vi "configuration UI.vi"() -> ()   [LabVIEW 2013]
uses:
  fixed channel editor.lvclass
  <vilib>/NI/Tag Bus Module Framework/channel/TBM channel.lvclass
  <vilib>/NI/Module Execution Interface/Engine Configuration/engine configuration.lvclass
  <vilib>/NI/Tag Bus/tag/tag descriptor.lvclass
  <vilib>/NI/Configuration Framework/Controls/EventCluster.ctl
  <vilib>/NI/Configuration Framework/NISE_CEF_TreeControl.lvlib
  <vilib>/NI/Tag Bus Data Framework/Configuration Editor/Classes/Engine Parent/Engine Parent Editor Node.lvclass
  <vilib>/NI/Tag Bus Module Framework/module configuration/TBM module configuration.lvclass
  <vilib>/NI/Tag Bus Data Framework/Configuration Editor/Classes/Module editor node/module editor node.lvclass
  module/configuration/fixed channel configuration.lvclass
  <vilib>/NI/Tag Bus Module Framework/channel/channel classification.ctl
  <vilib>/NI/Tools/Keyed Array/KeyedArray.ctl
  <vilib>/NI/Tools/Keyed Array/Tools_KeyedArray.lvlib
  <vilib>/NI/AMC/Message.ctl
  <vilib>/NI/AMC/AMC.lvlib
  <vilib>/NI/AMC/Message Queue.ctl
  <vilib>/NI/Configuration Framework/Node/NISE_CEF_Node.lvclass
  <vilib>/NI/Configuration Framework/Node/NodeRef.ctl
  <vilib>/NI/Configuration Framework/Node/UserEventRef.ctl
panel:
  in  "Tab Control":enum32{"Channels", "Parameters"}(tab)
  in  "mapwriters":bool
  out "Channel List":string[][](table)
  in  "mapall":bool
  in  "kvp":i32(listbox)
  in  "user event":T1
  in  "main queue":T2
  in  "node ref":T3
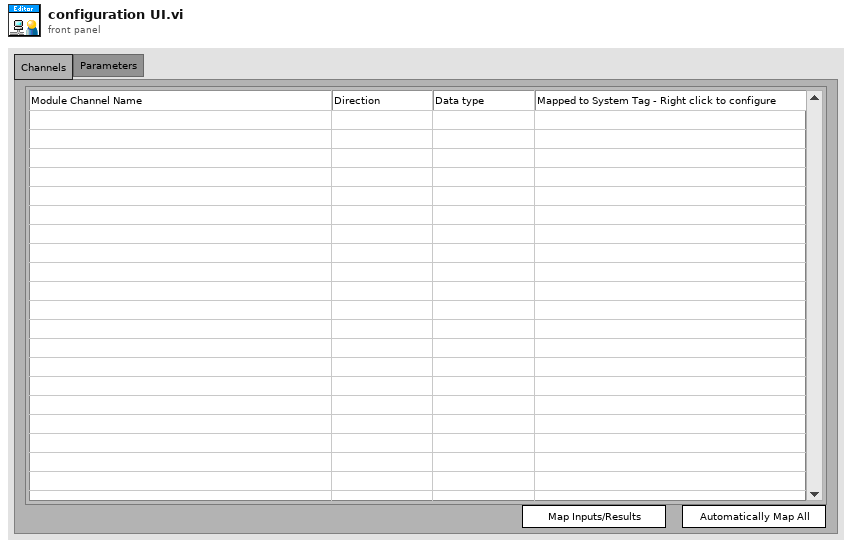
[diagram p1: front panel]
types:
  T1 = typedef "NISE_CEF_Node.lvclass/UserEventRef.ctl" = refnum<user-event>
  T2 = typedef "AMC.lvlib/Message Queue.ctl" = refnum<queue>
  T3 = typedef "NISE_CEF_Node.lvclass/NodeRef.ctl" = refnum<data-value>
  T4 = typedef "NISE_CEF_TreeControl.lvlib/EventCluster.ctl" = cluster{"command":string, "data":string}
  T5 = typedef "LVPoint32TypeDef.ctl" = cluster{"Horizontal":i32, "Vertical":i32}
  T6 = typedef "LVRowAndColumnTypeDef.ctl" = cluster{"Row":i32, "Column":i32}
  T7 = typedef "TBM channel.lvclass/channel classification.ctl" = enum16{"input data", "output data", "processing parameter", "processing result"}
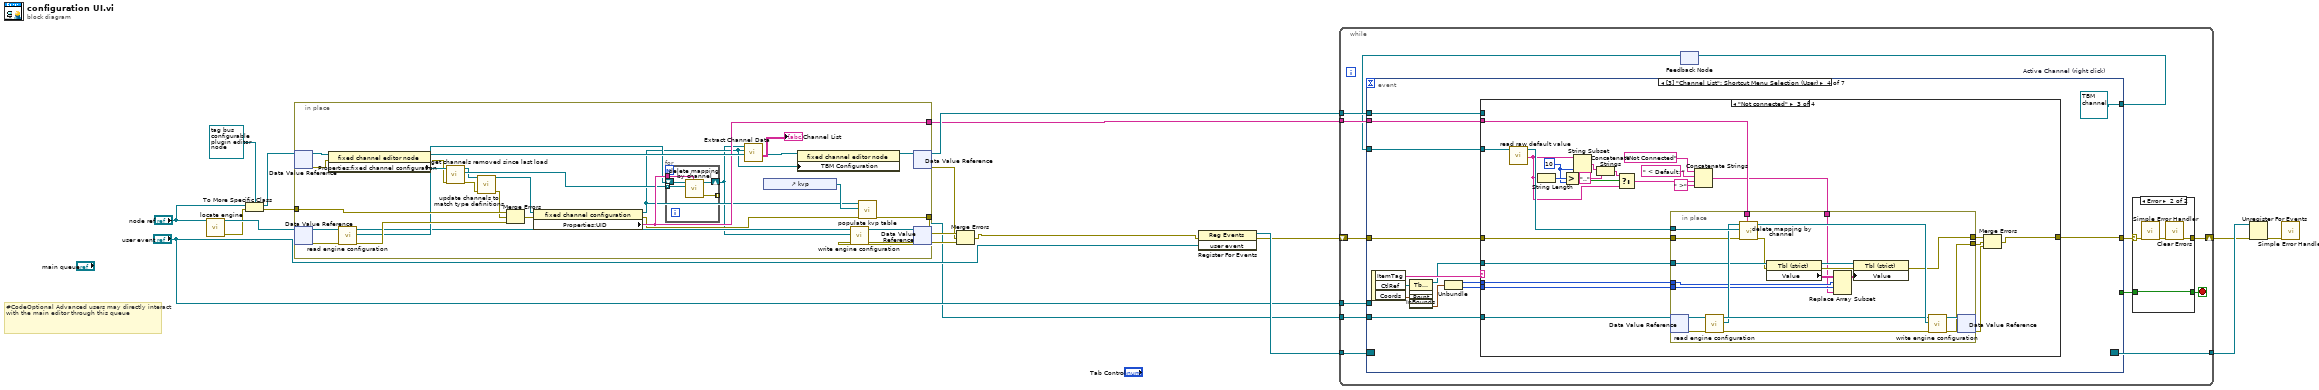
[diagram p0: block diagram]
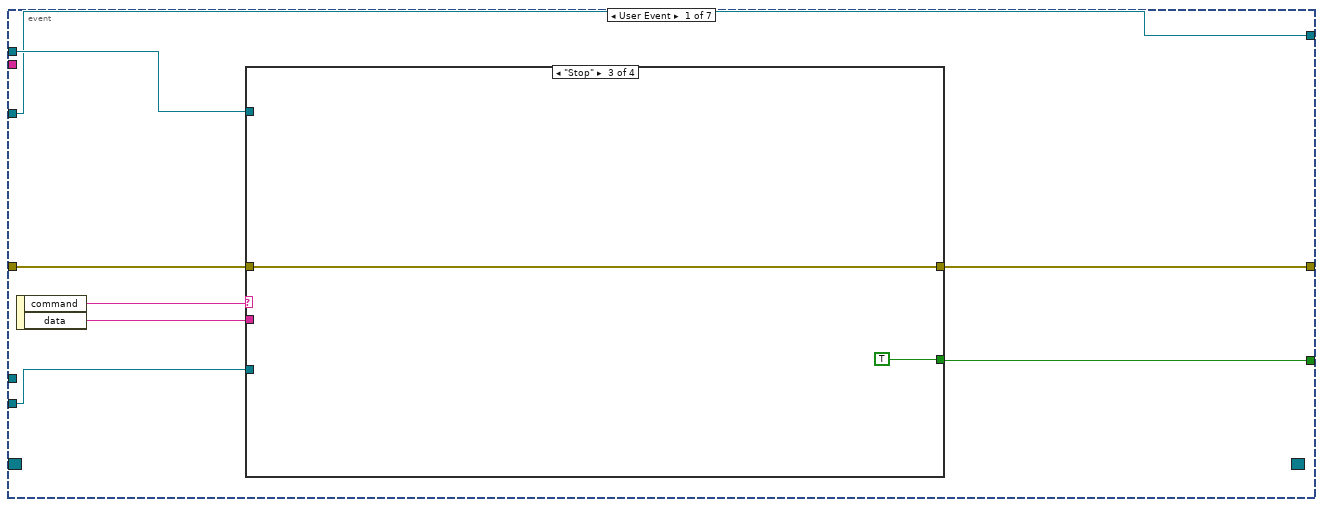
[diagram p3: hidden frame]
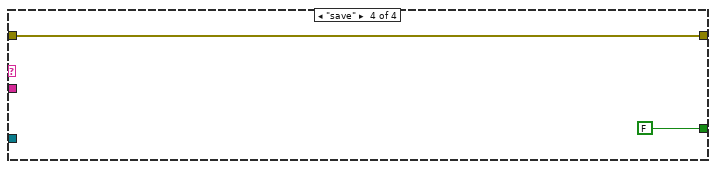
[diagram p6: hidden frame]
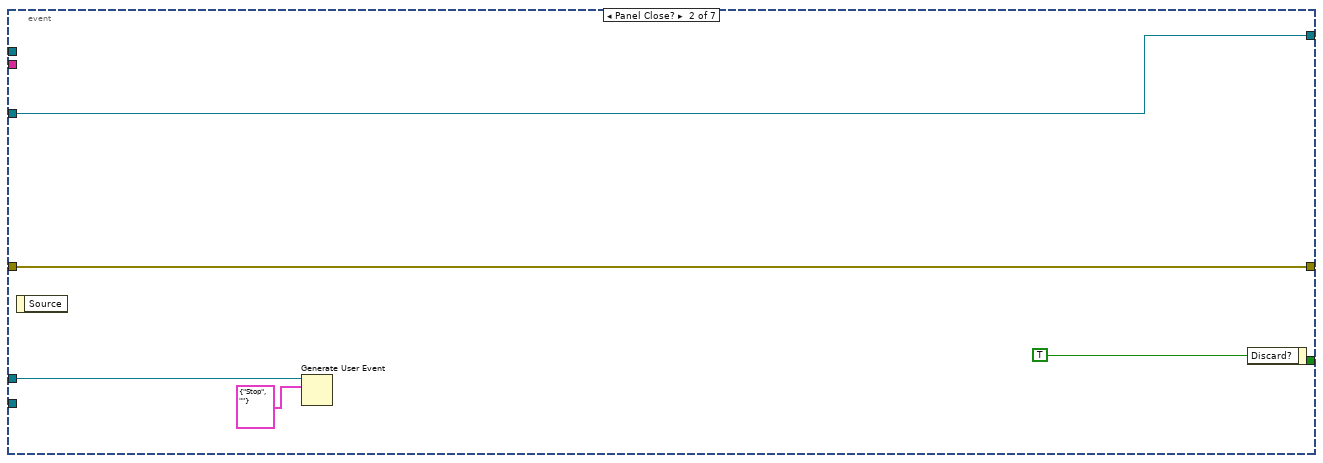
[diagram p7: hidden frame]
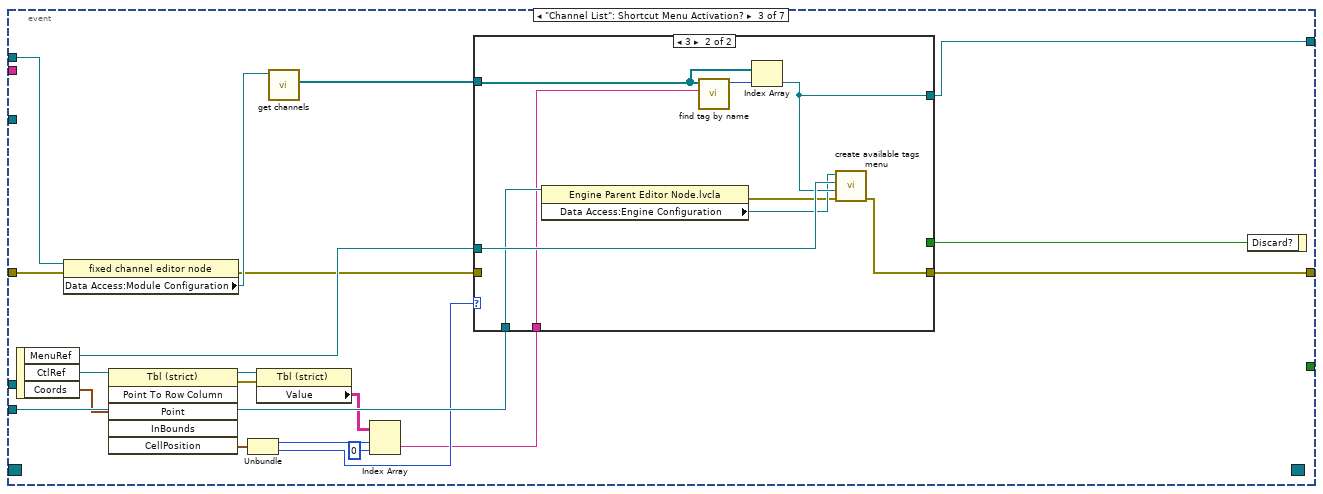
[diagram p8: hidden frame]
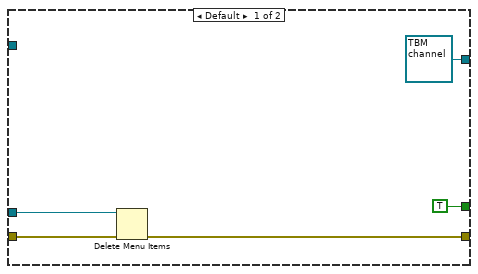
[diagram p9: hidden frame]
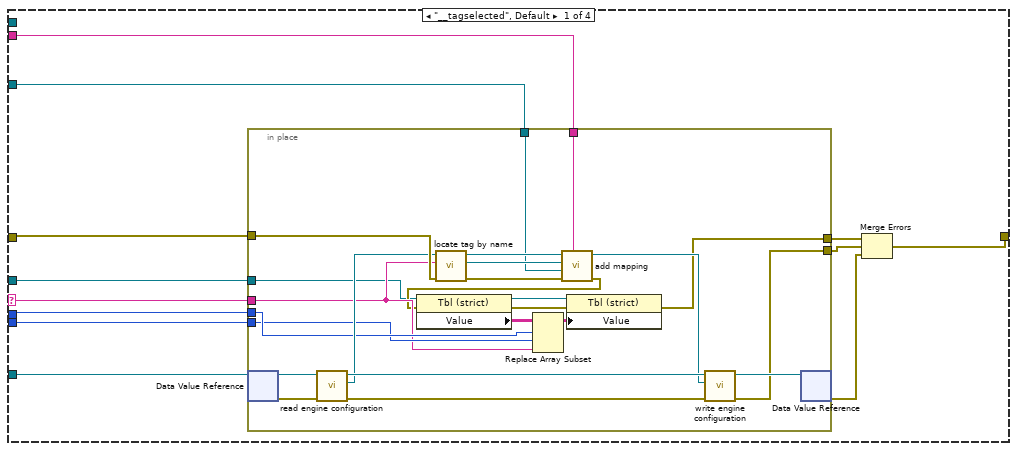
[diagram p10: hidden frame]
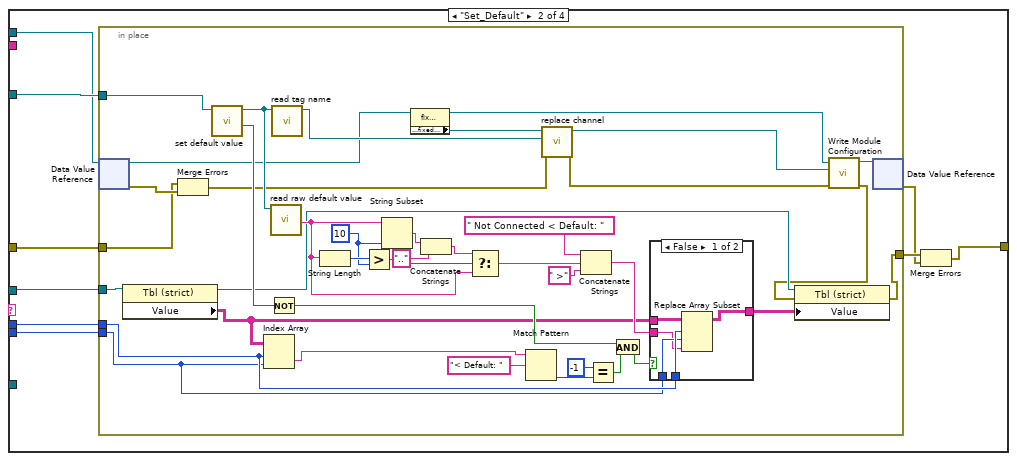
[diagram p11: hidden frame]
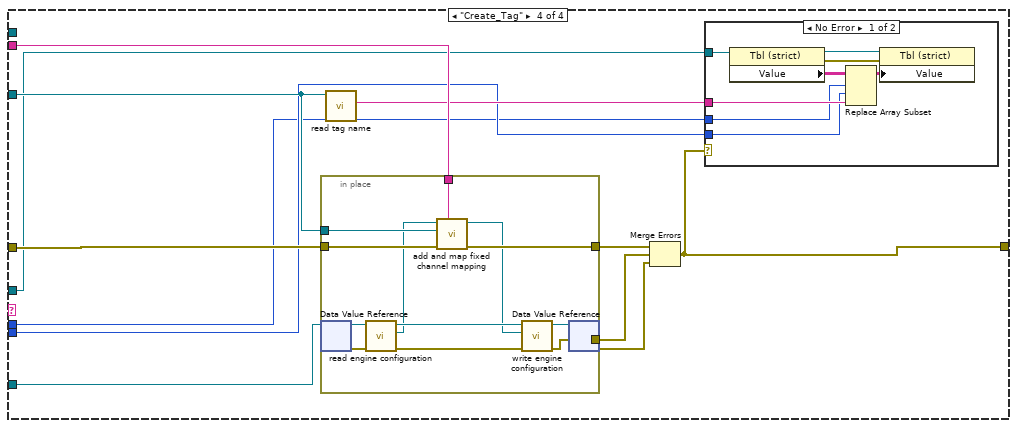
[diagram p13: hidden frame]
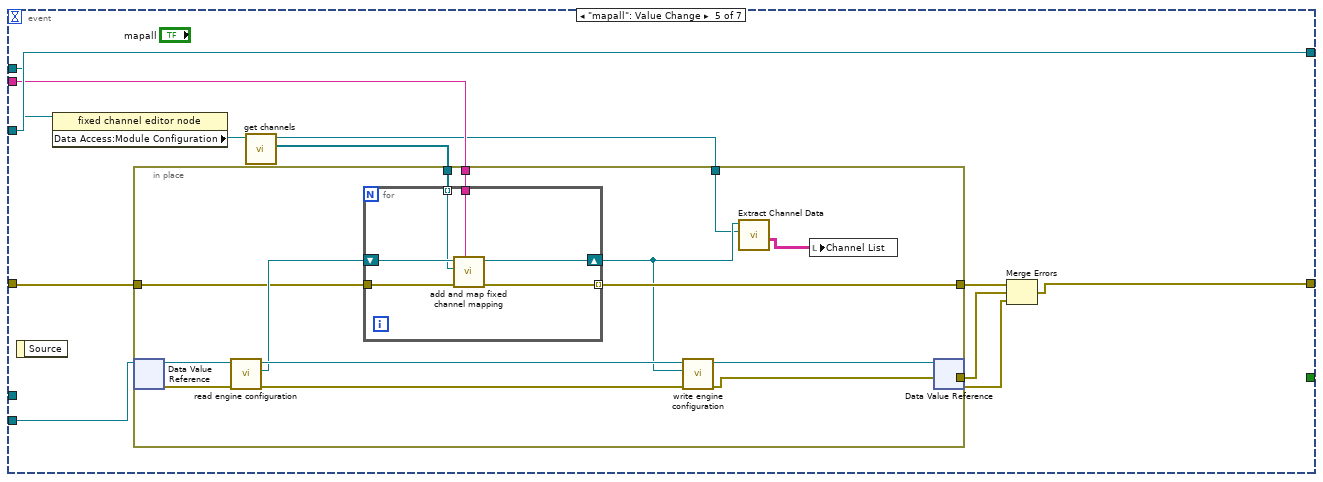
[diagram p15: hidden frame]
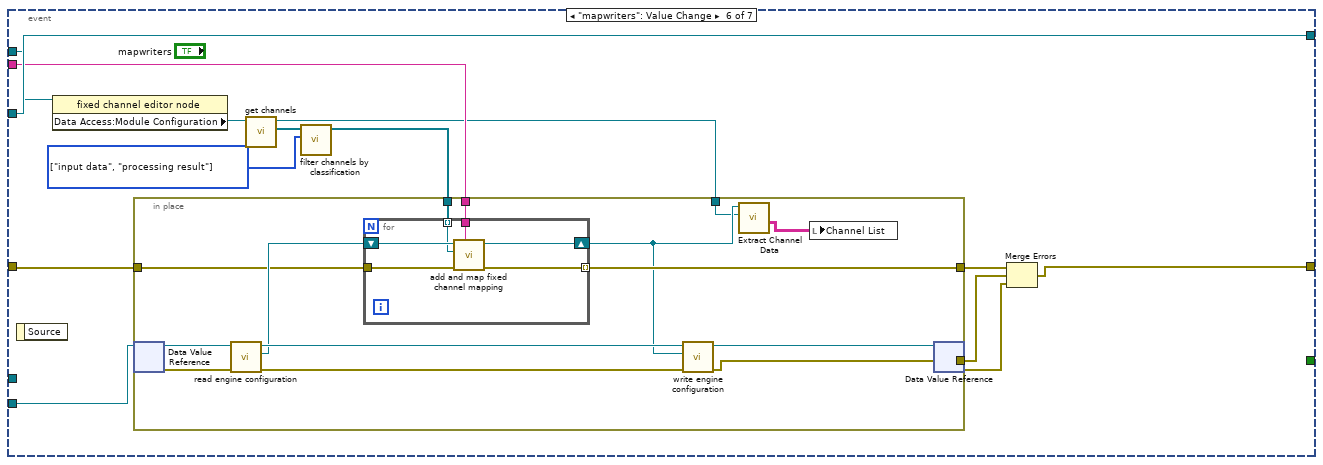
[diagram p16: hidden frame]
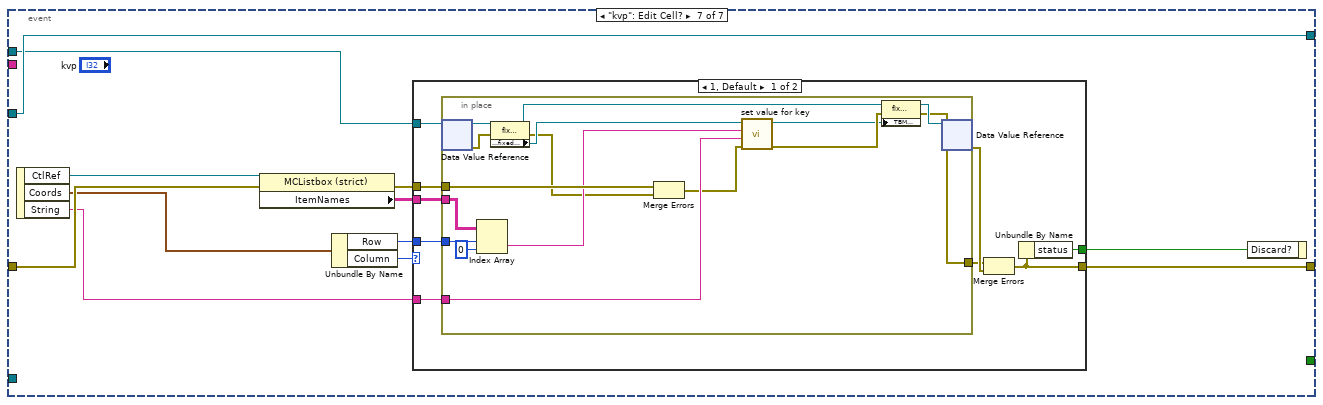
[diagram p17: hidden frame]
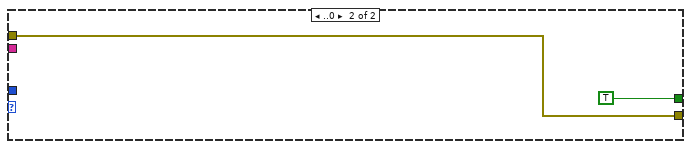
[diagram p18: hidden frame]
diagram:
  # "#CodeOptional Advanced users may directly interact with the main editor through this queue"
  n1 = call <vilib>:"locate engine.vi"("component"="node ref") -> ("error out"=w1:errorcluster, "engine"=w3:refnum<data-value>)  [unwired: 9 in]
  n2 = To More Specific Class(target class=refnum<data-value> refnum ("data value reference"), reference="node ref", error in=w1) -> (specific class reference=w12:refnum<data-value>, error out=w10:errorcluster)
  n3 = in-place {
    in-place-border: w10 -> [w45]
    in-place-border: [w38] -> w9
    in-place-border: [w33] -> w5
    n4 = in-place-dvr #1(w12) -> (w43:refnum<class "fixed channel editor.lvclass">, w35:errorcluster)
    n5 = in-place-dvr #2(w3) -> (w44:refnum<class "Engine Parent Editor Node.lvclass">, w39:errorcluster)
    n6 = property class="fixed channel editor node"(reference=w43, error in=w35) -> (reference out=w36:refnum<class "fixed channel editor.lvclass">, error out=w26:errorcluster, "Properties:fixed channel configuration"=w34:refnum<class "fixed channel configuration.lvclass">)
    n7 = call <vilib>:"read engine configuration.vi"("error in"=w39, "Engine Parent Editor Node in"=w44) -> ("error out"=w40:errorcluster, "engine configuration"=w31:refnum<class "engine configuration.lvclass">, "Engine Parent Editor Node out"=w22:refnum<class "Engine Parent Editor Node.lvclass">)  [unwired: 7 in]
    n8 = call "get channels removed since last load.vi"("error in"=w26, "fixed channel configuration in"=w34) -> ("error out"=w27:errorcluster, "removed"=w32:refnum<class "TBM channel.lvclass">[], "fixed channel configuration out"=w29:refnum<class "fixed channel configuration.lvclass">)  [unwired: 7 in]
    n9 = call "update channels to match type definitions.vi"("error in"=w27, "fixed channel configuration in"=w29) -> ("error out"=w25:errorcluster, "fixed channel configuration out"=w28:refnum<class "fixed channel configuration.lvclass">)  [unwired: 8 in]
    n10 = Merge Errors(w45, w25, w40) -> (w42:errorcluster)
    n11 = property class="fixed channel configuration"(reference=w28, error in=w42) -> (reference out=w23:refnum<class "fixed channel configuration.lvclass">, error out=w30:errorcluster, "Properties:UID"=w33:string)
    n12 = for {
      tunnel: w33 -> [w50]
      tunnel: w32 -> [w49] mode=indexing
      shift-right: [w48] -> w20
      shift-left: w31 -> [w47]
      tunnel: [w46] -> _ mode=indexing
      n13 = call <vilib>:"delete mapping by channel.vi"("owner ID"=w50, "channel"=w49, "engine configuration in"=w47) -> ("error out"=w46:errorcluster, "engine configuration out"=w48:refnum<class "engine configuration.lvclass">)  [unwired: 7 in]
    }
    n14 = call "Extract Channel Data.vi"("module configuration in"=w23, "Engine Configuration"=w20) -> ("Channel Data"=→"Channel List":string[][])  [unwired: 9 in]
    n15 = control-ref of="kvp"() -> (w37:refnum<vi>)
    n16 = property class="fixed channel editor node"(reference=w36, "TBM Configuration"=w23) -> (reference out=w24:refnum<class "fixed channel editor.lvclass">)  [unwired: 1 in, 1 out]
    n17 = call <vilib>:"write engine configuration.vi"("engine configuration"=w20, "Engine Parent Editor Node in"=w22) -> ("Engine Parent Editor Node out"=w21:refnum<class "Engine Parent Editor Node.lvclass">)  [unwired: 8 in, 1 out]
    n18 = call "populate kvp table.vi"("error in"=w30, "MCListbox Refnum"=w37, "fixed channel configuration in"=w23) -> ("error out"=w38:errorcluster)  [unwired: 8 in]
    n19 = in-place-dvr #1(w24) -> (w11:refnum<data-value>, w7:errorcluster)
    n20 = in-place-dvr #2(w21) -> (w6:refnum<data-value>, w8:errorcluster)
  }
  n21 = Merge Errors(w9, w7, w8) -> (w4:errorcluster)
  n22 = register-events(error in=w4, "user event") -> (reference out=w19:refnum<event-registration>, error out=w15:errorcluster)  [unwired: 1 in]
  n23 = while {
    tunnel: w19 -> [w63]
    tunnel: [w62] -> w18
    shift-right: [w58] -> w17
    shift-left: w15 -> [w61]
    tunnel: w5 -> [w57]
    tunnel: w11 -> [w56]
    tunnel: w6 -> [w55]
    tunnel: "user event" -> [w52]
    stop <- w59 stop-if-true
    n24 = feedback #3 "Active Channel (right click)"() -> (w53:refnum<class "TBM channel.lvclass">)  [unwired: 1 in]
    n25 = event shown="[3] \"Channel List\": Shortcut Menu Selection (User)" {
      selector: w63 -> [_ _ _ _ _ _ _]
      dyn-events: [_ _ _ _ _ _ _] -> w62
      timeout: _ -> [_ _ _ _ _ _ _]
      tunnel: [w76 _ _ _ _ _ _] -> w51
      tunnel: [w77 w88 w90 w132 w305 w340 w375] -> w60
      tunnel: w61 -> [w71 w88 w108 w133 w309 w343 w379]
      tunnel: w57 -> [_ _ _ w131 w314 w348 _]
      tunnel: w56 -> [w74 _ w105 w129 w308 w342 w371]
      tunnel: w55 -> [w73 _ w106 w130 w310 w344 _]
      tunnel: w53 -> [w70 w87 _ w134 w315 w349 w381]
      tunnel: [w70 w87 w107 refnum<class "TBM channel.lvclass"> refnum ("channel") w315 w349 w381] -> w54
      tunnel: w52 -> [_ w85 _ _ _ _ _]
      event User Event {
        n26 = event-data() -> ("command"=w75:string, "data"=w72:string)  [unwired: 1 in]
        n27 = case shown="\"Stop\"" w75 {
          tunnel: [_ _ TRUE FALSE] -> w76
          tunnel: w73 -> [_ _ _ _]
          tunnel: w71 -> [w78 w79 w80 w82]
          tunnel: [w78 w79 w80 w82] -> w77
          tunnel: w74 -> [_ _ _ _]
          tunnel: w72 -> [_ _ _ _]
          frame Default {
          }
          frame "Refresh" {
          }
          frame "Stop" {
          }
          frame "save" {
          }
        }
      }
      event Panel Close? {
        n28 = event-data() -> ()  [unwired: 1 in, 1 out]
        n29 = Generate User Event(user event=w85, event data cluster=T4 {"command"="Stop", "data"=""} ("event data")) -> ()  [unwired: 2 in, 2 out]
        n30 = event-data("Discard?"=TRUE) -> ()  [unwired: 1 in, 1 out]
      }
      event "Channel List": Shortcut Menu Activation? {
        n31 = event-data() -> ("MenuRef"=w101:refnum<k9>, "CtlRef"=w102:refnum<vi>, "Coords"=w100:T5)  [unwired: 1 in]
        n32 = property class="fixed channel editor node"(reference=w105, error in=w108) -> (error out=w91:errorcluster, "Data Access:Module Configuration"=w104:refnum<class "TBM module configuration.lvclass">)  [unwired: 1 out]
        n33 = invoke class="Tbl (strict)" method="Point To Row Column"(reference=w102, "Point"=w100) -> (reference out=w98:refnum<vi>, error out=w97:errorcluster, "CellPosition"=w99:T6)  [unwired: 4 in, 3 out]
        n34 = Unbundle(w99) -> ("Row"=w95:i32, "Column"=w93:i32)
        n35 = property class="Tbl (strict)"(reference=w98, error in=w97) -> ("Value"=w96:string[][])  [unwired: 2 out]
        n36 = call-dynamic "get channels.vi"("module configuration in"=w104) -> ("channels"=w103:refnum<class "TBM channel.lvclass">[])  [unwired: 9 in, 1 out]
        n37 = Index Array(array=w96, index (row)=w95, index (col)=0 ("disabled index (col)")) -> (element=w92:string)
        n38 = case shown="3" w93 {
          tunnel: w101 -> [w112 w122]
          tunnel: [w110 w114] -> w90
          tunnel: w103 -> [_ w116]
          tunnel: [refnum<class "TBM channel.lvclass"> refnum ("channel") w121] -> w107
          tunnel: w106 -> [_ w119]
          tunnel: w92 -> [_ w117]
          tunnel: w91 -> [w111 _]
          tunnel: [TRUE _] -> w89
          frame Default {
            n39 = Delete Menu Items(6:w111, 9:w112) -> (0:w110:errorcluster)  [unwired: 2 in, 1 out]
          }
          frame 3 {
            n40 = property class="Engine Parent Editor Node.lvcla"(reference=w119) -> (error out=w115:errorcluster, "Data Access:Engine Configuration"=w118:refnum<class "engine configuration.lvclass">)  [unwired: 1 in, 1 out]
            n41 = call <vilib>:"find tag by name.vi"("name"=w117, "tags in"=w116) -> ("index"=w120:i32)  [unwired: 9 in]
            n42 = Index Array(array=w116, index=w120) -> (element=w121:refnum<class "TBM channel.lvclass">)
            n43 = call "create available tags menu.vi"("error in"=w115, "channel to map to"=w121, "MenuRef"=w122, "engine configuration in"=w118) -> ("error out"=w114:errorcluster)  [unwired: 6 in, 1 out]
          }
        }
        n44 = event-data("Discard?"=w89) -> ()  [unwired: 1 in, 1 out]
      }
      event "Channel List": Shortcut Menu Selection (User) {
        n45 = event-data() -> ("ItemTag"=w136:string, "CtlRef"=w128:refnum<vi>, "Coords"=w127:T5)  [unwired: 1 in]
        n46 = invoke class="Tbl (strict)" method="Point To Row Column"(reference=w128, "Point"=w127) -> (reference out=w123:refnum<vi>, "CellPosition"=w126:T6)  [unwired: 4 in, 4 out]
        n47 = Unbundle(w126) -> ("Row"=w125:i32, "Column"=w124:i32)
        n48 = case shown="\"Not connected\"" w136 {
          selector: w136 -> [w146 _ _ _]
          tunnel: w124 -> [w148 w180 w250 w274]
          tunnel: w125 -> [w147 w179 w249 w273]
          tunnel: w134 -> [w144 w181 w245 w277]
          tunnel: [w141 w177 w230 w275] -> w132
          tunnel: w133 -> [w145 w173 w248 w283]
          tunnel: w131 -> [w142 _ w246 w281]
          tunnel: w130 -> [w138 _ w231 w280]
          tunnel: w129 -> [_ w178 _ _]
          tunnel: w123 -> [w137 w174 w227 w272]
          frame "__tagselected", Default {
            n49 = in-place {
              in-place-border: w148 -> [w153]
              in-place-border: w147 -> [w154]
              in-place-border: w146 -> [w152]
              in-place-border: w145 -> [w172]
              in-place-border: w144 -> [w169]
              in-place-border: [w150] -> w143
              in-place-border: w142 -> [w167]
              in-place-border: [w161] -> w139
              in-place-border: w137 -> [w149]
              n50 = in-place-dvr #4(w138) -> (w164:refnum<class "Engine Parent Editor Node.lvclass">, w163:errorcluster)
              n51 = call <vilib>:"read engine configuration.vi"("error in"=w163, "Engine Parent Editor Node in"=w164) -> ("error out"=w165:errorcluster, "engine configuration"=w159:refnum<class "engine configuration.lvclass">, "Engine Parent Editor Node out"=w166:refnum<class "Engine Parent Editor Node.lvclass">)  [unwired: 7 in]
              n52 = call <vilib>:"locate tag by name.vi"("error in"=w172, "tag name"=w152, "engine configuration in"=w159) -> ("error out"=w168:errorcluster, "tag descriptor"=w170:refnum<class "tag descriptor.lvclass">, "engine configuration out"=w171:refnum<class "engine configuration.lvclass">)  [unwired: 6 in]
              n53 = call <vilib>:"add mapping.vi"("owner ID"=w167, "error in"=w168, "channel"=w169, "tag descriptor"=w170, "engine configuration"=w171) -> ("error out"=w151:errorcluster, "engine configuration out"=w160:refnum<class "engine configuration.lvclass">)  [unwired: 5 in]
              n54 = property class="Tbl (strict)"(reference=w149, error in=w151) -> (reference out=w156:refnum<vi>, error out=w157:errorcluster, "Value"=w155:string[][])
              n55 = Replace Array Subset(array=w155, new element=w152, index (row)=w154, index (col)=w153) -> (w158:string[][])
              n56 = property class="Tbl (strict)"(reference=w156, error in=w157, "Value"=w158) -> (error out=w150:errorcluster)  [unwired: 1 out]
              n57 = call <vilib>:"write engine configuration.vi"("error in"=w165, "engine configuration"=w160, "Engine Parent Editor Node in"=w166) -> ("error out"=w161:errorcluster, "Engine Parent Editor Node out"=w162:refnum<class "Engine Parent Editor Node.lvclass">)  [unwired: 7 in]
              n58 = in-place-dvr #4(w162) -> (w140:errorcluster)  [unwired: 1 out]
            }
            n59 = Merge Errors(w143, w139, w140) -> (w141:errorcluster)
          }
          frame "Set_Default" {
            n60 = in-place {
              in-place-border: w181 -> [w220]
              in-place-border: w180 -> [w189]
              in-place-border: w179 -> [w190]
              in-place-border: [w187] -> w176
              in-place-border: w174 -> [w195]
              in-place-border: w173 -> [w182]
              w209 = 10 ("y")
              n61 = in-place-dvr #5(w178) -> (w185:refnum<class "fixed channel editor.lvclass">, w198:errorcluster)
              n62 = property class="Tbl (strict)"(reference=w195) -> (reference out=w193:refnum<vi>, "Value"=w192:string[][])  [unwired: 1 in, 1 out]
              n63 = Merge Errors(w182, w198) -> (w183:errorcluster)
              n64 = call "set default value.vi"("tag"=w220) -> ("cancelled?"=w212:bool, "tag out"=w204:refnum<class "TBM channel.lvclass">)  [unwired: 9 in]
              n65 = Index Array(array=w192, index (row)=w190, index (col)=w189) -> (element=w191:string)
              n66 = Not(x=w212) -> (.not. x?=w201:bool)
              n67 = call <vilib>:"read raw default value.vi"("system tag in"=w204) -> ("raw default"=w205:string)  [unwired: 8 in, 2 out]
              n68 = call <vilib>:"read tag name.vi"("system tag in"=w204) -> ("system tag out"=w196:refnum<class "TBM channel.lvclass">)  [unwired: 8 in, 2 out]
              n69 = String Length(string=w205) -> (length=w211:i32)
              n70 = Greater?(x=w211, y=w209) -> (0:w210:bool)
              n71 = String Subset(string=w205, length (rest)=w209) -> (substring=w207:string)  [unwired: 1 in]
              n72 = property class="fixed channel editor node"(reference=w185) -> (reference out=w184:refnum<class "fixed channel editor.lvclass">, "Properties:fixed channel configuration"=w186:refnum<class "fixed channel configuration.lvclass">)  [unwired: 1 in, 1 out]
              n73 = Concatenate Strings(w207, ".." ("string")) -> (w208:string)
              n74 = Select(t=w208, s=w210, f=w205) -> (s? t:f=w203:string)
              n75 = Match Pattern(string=w191, regular expression="< Default: ") -> (offset past match=w218:i32)  [unwired: 1 in, 3 out]
              n76 = call "replace channel.vi"("error in"=w183, "channel"=w196, "fixed module parent implementation configuration in"=w186) -> ("error out"=w197:errorcluster, "fixed module parent implementation configuration out"=w199:refnum<class "fixed channel configuration.lvclass">)  [unwired: 7 in]
              n77 = Concatenate Strings(" Not Connected < Default: " ("string"), w203, " >" ("string")) -> (w202:string)
              n78 = Equal?(x=-1, y=w218) -> (x = y?=w216:bool)
              n79 = And(x=w201, y=w216) -> (x .and. y?=w213:bool)
              n80 = case shown="False" w213 {
                tunnel: w202 -> [w221 _]
                tunnel: w192 -> [w225 w226]
                tunnel: [w224 w226] -> w194
                tunnel: w190 -> [w223 _]
                tunnel: w189 -> [w222 _]
                frame False {
                  n81 = Replace Array Subset(array=w225, new element=w221, index (row)=w223, index (col)=w222) -> (w224:string[][])
                }
                frame True {
                }
              }
              n82 = call <vilib>:"Write Module Configuration.vi"("error in"=w197, "module configuration"=w199, "Module Editor Node in"=w184) -> ("error out"=w188:errorcluster, "Module Editor Node out"=w200:refnum<class "fixed channel editor.lvclass">)  [unwired: 7 in]
              n83 = property class="Tbl (strict)"(reference=w193, error in=w188, "Value"=w194) -> (error out=w187:errorcluster)  [unwired: 1 out]
              n84 = in-place-dvr #5(w200) -> (w175:errorcluster)  [unwired: 1 out]
            }
            n85 = Merge Errors(w176, w175) -> (w177:errorcluster)
          }
          frame "Not connected" {
            w238 = 10 ("y")
            n86 = call <vilib>:"read raw default value.vi"("system tag in"=w245) -> ("raw default"=w234:string, "system tag out"=w244:refnum<class "TBM channel.lvclass">)  [unwired: 8 in, 1 out]
            n87 = String Length(string=w234) -> (length=w240:i32)
            n88 = Greater?(x=w240, y=w238) -> (0:w239:bool)
            n89 = String Subset(string=w234, length (rest)=w238) -> (substring=w236:string)  [unwired: 1 in]
            n90 = Concatenate Strings(w236, ".." ("string")) -> (w237:string)
            n91 = Select(t=w237, s=w239, f=w234) -> (s? t:f=w233:string)
            n92 = Concatenate Strings("Not Connected" ("string"), " < Default: " ("string"), w233, " >" ("string")) -> (w243:string)
            n93 = in-place {
              in-place-border: w250 -> [w256]
              in-place-border: w249 -> [w257]
              in-place-border: w248 -> [w253]
              in-place-border: [w251] -> w247
              in-place-border: w246 -> [w271]
              in-place-border: w244 -> [w270]
              in-place-border: w243 -> [w254]
              in-place-border: [w265] -> w228
              in-place-border: w227 -> [w255]
              n94 = in-place-dvr #6(w231) -> (w269:refnum<class "Engine Parent Editor Node.lvclass">, w268:errorcluster)
              n95 = call <vilib>:"read engine configuration.vi"("error in"=w268, "Engine Parent Editor Node in"=w269) -> ("error out"=w266:errorcluster, "engine configuration"=w262:refnum<class "engine configuration.lvclass">, "Engine Parent Editor Node out"=w263:refnum<class "Engine Parent Editor Node.lvclass">)  [unwired: 7 in]
              n96 = call <vilib>:"delete mapping by channel.vi"("owner ID"=w271, "error in"=w253, "channel"=w270, "engine configuration in"=w262) -> ("error out"=w252:errorcluster, "engine configuration out"=w264:refnum<class "engine configuration.lvclass">)  [unwired: 6 in]
              n97 = property class="Tbl (strict)"(reference=w255, error in=w252) -> (reference out=w259:refnum<vi>, error out=w260:errorcluster, "Value"=w258:string[][])
              n98 = Replace Array Subset(array=w258, new element=w254, index (row)=w257, index (col)=w256) -> (w261:string[][])
              n99 = property class="Tbl (strict)"(reference=w259, error in=w260, "Value"=w261) -> (error out=w251:errorcluster)  [unwired: 1 out]
              n100 = call <vilib>:"write engine configuration.vi"("error in"=w266, "engine configuration"=w264, "Engine Parent Editor Node in"=w263) -> ("error out"=w265:errorcluster, "Engine Parent Editor Node out"=w267:refnum<class "Engine Parent Editor Node.lvclass">)  [unwired: 7 in]
              n101 = in-place-dvr #6(w267) -> (w229:errorcluster)  [unwired: 1 out]
            }
            n102 = Merge Errors(w247, w228, w229) -> (w230:errorcluster)
          }
          frame "Create_Tag" {
            n103 = in-place {
              in-place-border: w283 -> [w303]
              in-place-border: [w302] -> w282
              in-place-border: w281 -> [w301]
              in-place-border: w277 -> [w300]
              in-place-border: [w296] -> w278
              n104 = in-place-dvr #7(w280) -> (w298:refnum<class "Engine Parent Editor Node.lvclass">, w299:errorcluster)
              n105 = call <vilib>:"read engine configuration.vi"("error in"=w299, "Engine Parent Editor Node in"=w298) -> ("error out"=w295:errorcluster, "engine configuration"=w293:refnum<class "engine configuration.lvclass">, "Engine Parent Editor Node out"=w294:refnum<class "Engine Parent Editor Node.lvclass">)  [unwired: 7 in]
              n106 = call <vilib>:"add and map fixed channel mapping.vi"("module instance"=w301, "error in"=w303, "fixed channel"=w300, "engine configuration in"=w293) -> ("error out"=w302:errorcluster, "engine configuration out"=w292:refnum<class "engine configuration.lvclass">)  [unwired: 6 in]
              n107 = call <vilib>:"write engine configuration.vi"("error in"=w295, "engine configuration"=w292, "Engine Parent Editor Node in"=w294) -> ("error out"=w296:errorcluster, "Engine Parent Editor Node out"=w297:refnum<class "Engine Parent Editor Node.lvclass">)  [unwired: 7 in]
              n108 = in-place-dvr #7(w297) -> (w279:errorcluster)  [unwired: 1 out]
            }
            n109 = call <vilib>:"read tag name.vi"("system tag in"=w277) -> ("name"=w276:string)  [unwired: 8 in, 2 out]
            n110 = Merge Errors(w282, w278, w279) -> (w275:errorcluster)
            n111 = case shown="No Error" w275 {
              tunnel: w276 -> [w287 _]
              tunnel: w274 -> [w286 _]
              tunnel: w273 -> [w285 _]
              tunnel: w272 -> [w284 _]
              frame No Error {
                n112 = property class="Tbl (strict)"(reference=w284) -> (reference out=w289:refnum<vi>, error out=w290:errorcluster, "Value"=w288:string[][])  [unwired: 1 in]
                n113 = Replace Array Subset(array=w288, new element=w287, index (row)=w285, index (col)=w286) -> (w291:string[][])
                n114 = property class="Tbl (strict)"(reference=w289, error in=w290, "Value"=w291) -> ()  [unwired: 2 out]
              }
              frame Error {
              }
            }
          }
        }
      }
      event "mapall": Value Change {
        n115 = event-data() -> ()  [unwired: 1 in, 1 out]
        n116 = property class="fixed channel editor node"(reference=w308) -> ("Data Access:Module Configuration"=w307:refnum<class "TBM module configuration.lvclass">)  [unwired: 1 in, 2 out]
        n117 = call-dynamic "get channels.vi"("module configuration in"=w307) -> ("channels"=w306:refnum<class "TBM channel.lvclass">[], "module configuration out"=w304:refnum<class "TBM module configuration.lvclass">)  [unwired: 9 in]
        n118 = in-place {
          in-place-border: [w329] -> w313
          in-place-border: [w325] -> w312
          in-place-border: w314 -> [w321]
          in-place-border: w309 -> [w320]
          in-place-border: w306 -> [w319]
          in-place-border: w304 -> [w316]
          n119 = in-place-dvr #8(w310) -> (w327:refnum<class "Engine Parent Editor Node.lvclass">, w328:errorcluster)
          n120 = call <vilib>:"read engine configuration.vi"("error in"=w328, "Engine Parent Editor Node in"=w327) -> ("error out"=w324:errorcluster, "engine configuration"=w322:refnum<class "engine configuration.lvclass">, "Engine Parent Editor Node out"=w323:refnum<class "Engine Parent Editor Node.lvclass">)  [unwired: 7 in]
          n121 = for {
            tunnel: [w335] -> w329 mode=indexing
            tunnel: w321 -> [w332]
            tunnel: w320 -> [w331]
            shift-right: [w333] -> w317
            shift-left: w322 -> [w334]
            tunnel: w319 -> [w330] mode=indexing
            n122 = call <vilib>:"add and map fixed channel mapping.vi"("module instance"=w332, "error in"=w331, "fixed channel"=w330, "engine configuration in"=w334) -> ("error out"=w335:errorcluster, "engine configuration out"=w333:refnum<class "engine configuration.lvclass">)  [unwired: 6 in]
          }
          n123 = call <vilib>:"write engine configuration.vi"("error in"=w324, "engine configuration"=w317, "Engine Parent Editor Node in"=w323) -> ("error out"=w325:errorcluster, "Engine Parent Editor Node out"=w326:refnum<class "Engine Parent Editor Node.lvclass">)  [unwired: 7 in]
          n124 = call "Extract Channel Data.vi"("module configuration in"=w316, "Engine Configuration"=w317) -> ("Channel Data"=w318:string[][])  [unwired: 9 in]
          n125 = local write "Channel List"(w318) -> ()
          n126 = in-place-dvr #8(w326) -> (w311:errorcluster)  [unwired: 1 out]
        }
        n127 = Merge Errors(w313, w312, w311) -> (w305:errorcluster)
      }
      event "mapwriters": Value Change {
        w338 = T7[] [enum."input data", enum."processing result"] items=["input data", "output data", "processing parameter", "processing result"] ("allowed classifications")
        n128 = event-data() -> ()  [unwired: 1 in, 1 out]
        n129 = property class="fixed channel editor node"(reference=w342) -> ("Data Access:Module Configuration"=w341:refnum<class "TBM module configuration.lvclass">)  [unwired: 1 in, 2 out]
        n130 = call-dynamic "get channels.vi"("module configuration in"=w341) -> ("channels"=w337:refnum<class "TBM channel.lvclass">[], "module configuration out"=w339:refnum<class "TBM module configuration.lvclass">)  [unwired: 9 in]
        n131 = call <vilib>:"filter channels by classification.vi"("allowed classifications"=w338, "channels in"=w337) -> ("channels out"=w336:refnum<class "TBM channel.lvclass">[])  [unwired: 9 in]
        n132 = in-place {
          in-place-border: [w363] -> w347
          in-place-border: [w359] -> w346
          in-place-border: w348 -> [w355]
          in-place-border: w343 -> [w354]
          in-place-border: w336 -> [w353]
          in-place-border: w339 -> [w350]
          n133 = in-place-dvr #9(w344) -> (w361:refnum<class "Engine Parent Editor Node.lvclass">, w362:errorcluster)
          n134 = call <vilib>:"read engine configuration.vi"("error in"=w362, "Engine Parent Editor Node in"=w361) -> ("error out"=w358:errorcluster, "engine configuration"=w356:refnum<class "engine configuration.lvclass">, "Engine Parent Editor Node out"=w357:refnum<class "Engine Parent Editor Node.lvclass">)  [unwired: 7 in]
          n135 = for {
            tunnel: [w369] -> w363 mode=indexing
            tunnel: w355 -> [w366]
            tunnel: w354 -> [w365]
            shift-right: [w367] -> w351
            shift-left: w356 -> [w368]
            tunnel: w353 -> [w364] mode=indexing
            n136 = call <vilib>:"add and map fixed channel mapping.vi"("module instance"=w366, "error in"=w365, "fixed channel"=w364, "engine configuration in"=w368) -> ("error out"=w369:errorcluster, "engine configuration out"=w367:refnum<class "engine configuration.lvclass">)  [unwired: 6 in]
          }
          n137 = call <vilib>:"write engine configuration.vi"("error in"=w358, "engine configuration"=w351, "Engine Parent Editor Node in"=w357) -> ("error out"=w359:errorcluster, "Engine Parent Editor Node out"=w360:refnum<class "Engine Parent Editor Node.lvclass">)  [unwired: 7 in]
          n138 = call "Extract Channel Data.vi"("module configuration in"=w350, "Engine Configuration"=w351) -> ("Channel Data"=w352:string[][])  [unwired: 9 in]
          n139 = local write "Channel List"(w352) -> ()
          n140 = in-place-dvr #9(w360) -> (w345:errorcluster)  [unwired: 1 out]
        }
        n141 = Merge Errors(w347, w346, w345) -> (w340:errorcluster)
      }
      event "kvp": Edit Cell? {
        n142 = event-data() -> ("CtlRef"=w380:refnum<vi>, "Coords"=w370:T6, "String"=w372:string)  [unwired: 1 in]
        n143 = property class="MCListbox (strict)"(reference=w380, error in=w379) -> (error out=w376:errorcluster, "ItemNames"=w374:string[][])  [unwired: 1 out]
        n144 = Unbundle By Name(w370) -> ("Row"=w373:i32, "Column"=w378:i32)
        n145 = case shown="1, Default" w378 {
          tunnel: [w386 TRUE] -> w377
          tunnel: w376 -> [w389 w407]
          tunnel: [w387 w407] -> w375
          tunnel: w374 -> [w385 _]
          tunnel: w373 -> [w384 _]
          tunnel: w372 -> [w383 _]
          tunnel: w371 -> [w390 _]
          frame 1, Default {
            n146 = in-place {
              in-place-border: w389 -> [w406]
              in-place-border: w385 -> [w405]
              in-place-border: w384 -> [w403]
              in-place-border: w383 -> [w401]
              in-place-border: [w391] -> w382
              n147 = in-place-dvr #10(w390) -> (w399:refnum<class "fixed channel editor.lvclass">, w397:errorcluster)
              n148 = Index Array(array=w405, index (row)=w403, index (col)=0 ("disabled index (col)")) -> (element=w402:string)
              n149 = property class="fixed channel editor node"(reference=w399, error in=w397) -> (reference out=w394:refnum<class "fixed channel editor.lvclass">, error out=w396:errorcluster, "Properties:fixed channel configuration"=w398:refnum<class "fixed channel configuration.lvclass">)
              n150 = Merge Errors(w406, w396) -> (w400:errorcluster)
              n151 = call-dynamic "set value for key.vi"("error in"=w400, "value"=w401, "key"=w402, "fixed channel configuration in"=w398) -> ("error out"=w395:errorcluster, "fixed channel configuration out"=w392:refnum<class "fixed channel configuration.lvclass">)  [unwired: 6 in]
              n152 = property class="fixed channel editor node"(reference=w394, error in=w395, "TBM Configuration"=w392) -> (reference out=w393:refnum<class "fixed channel editor.lvclass">, error out=w391:errorcluster)
              n153 = in-place-dvr #10(w393) -> (w388:errorcluster)  [unwired: 1 out]
            }
            n154 = Merge Errors(w382, w388) -> (w387:errorcluster)
            n155 = Unbundle By Name(w387) -> ("status"=w386:bool)
          }
          frame ..0 {
          }
        }
        n156 = event-data("Discard?"=w377) -> ()  [unwired: 1 in, 1 out]
      }
    }
    n157 = feedback-in #3(w54) -> ()
    n158 = case shown="Error" w60 {
      selector: w60 -> [w64 w67]
      tunnel: [w65 w69] -> w59
      tunnel: w51 -> [w65 w69]
      tunnel: [w64 w68] -> w58
      frame No Error {
      }
      frame Error {
        n159 = call <vilib>:"Simple Error Handler.vi"("error in (no error)"=w67) -> ("error out"=w66:errorcluster)  [unwired: 4 in, 4 out]
        n160 = call <vilib>:"Clear Errors.vi"("error in (no error)"=w66) -> ("error out"=w68:errorcluster)  [unwired: 6 in]
      }
    }
  }
  n161 = Unregister For Events(event registration refnum=w18, error in=w17) -> (error out=w14:errorcluster)
  n162 = call <vilib>:"Simple Error Handler.vi"("error in (no error)"=w14) -> ()  [unwired: 4 in, 5 out]
